vi "Name (offset).vi"(8 "error in (no error)":errorcluster, 10 "offset (0)":i32, 11 "JSON":string) -> (0 "error out":errorcluster, 1 "JSON name":string, 2 "offset":i32)   [LabVIEW 2020, in "Library Commun.lvlib" / "JSON Value.lvclass"]
doc: "Splits a JSON value string into a name and it's value. Unescapes the name.\n\nCopyright 2012 James David Powell, Shaun Rumbell and Ton Plomp\nMore information on http://lavag.org/topic/16217-cr-json-labview"
uses:
  JSON Value.lvclass
  JSON Scalar/Unescape JSON string.vi
  support/JSON support.lvlib
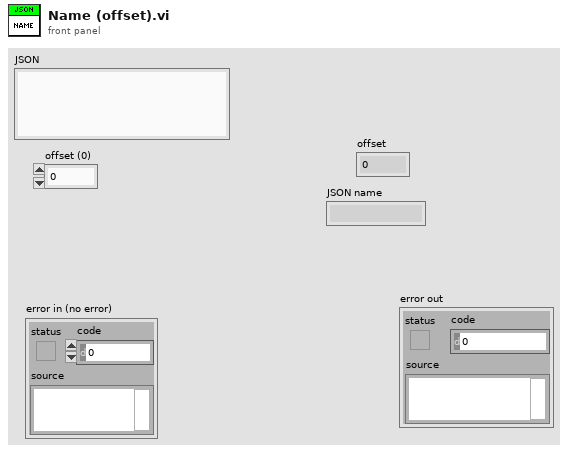
[diagram p1: front panel]
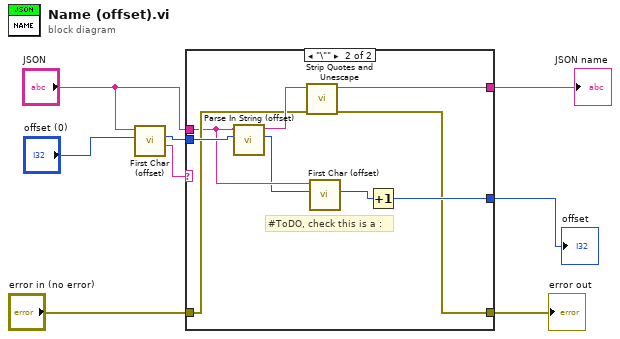
[diagram p0: block diagram]
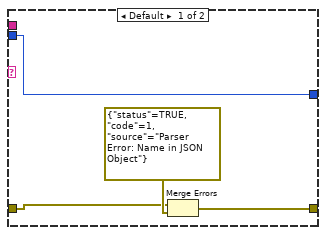
[diagram p2: hidden frame]
diagram:
  n1 = call "First Char (offset).vi"("offset (0)"="offset (0)", "String in"="JSON") -> ("First Char"=w5:string, "Offset"=w3:i32)  [unwired: 8 in]
  n2 = case shown="\"\\\"\"" w5 {
    tunnel: "JSON" -> [_ w16]
    tunnel: [_ w14] -> w8
    tunnel: [w10 w13] -> w7
    tunnel: "error in (no error)" -> [w11 w19]
    tunnel: w3 -> [w9 w20]
    tunnel: [w9 w17] -> w2
    frame Default {
      n3 = Merge Errors(w11, errorcluster {"status"=TRUE, "code"=1, "source"="Parser Error: Name in JSON Object"} ("error in")) -> (w10:errorcluster)
    }
    frame "\"" {
      # "#ToDO, check this is a :"
      n4 = call "Parse In String (offset).vi"("offset"=w20, "JSON (quote at offset)"=w16) -> ("offset"=w15:i32, "String (incl quotes)"=w21:string)  [unwired: 8 in]
      n5 = call "Strip Quotes and Unescape.vi"("error in (no error)"=w19, "String"=w21) -> ("error out"=w13:errorcluster, "result string"=w14:string)  [unwired: 7 in, 1 out]
      n6 = call "First Char (offset).vi"("offset (0)"=w15, "String in"=w16) -> ("Offset"=w18:i32)  [unwired: 8 in, 1 out]
      n7 = Increment(x=w18) -> (x+1=w17:i32)
    }
  }
  "JSON name" <- w8
  "error out" <- w7
  "offset" <- w2
